vi "TSCAN_Table.vi"(6 "Message Name":string[][](array[string]), 7 "ms?":bool, 8 "SigValue":dbl[][](array[numeric]), 9 "SigName":string[][](array[string]), 10 "Buffer":T1(array[cluster]), 11 "MCListbox reference handle":refnum<vi>) -> ()   [LabVIEW 2014]
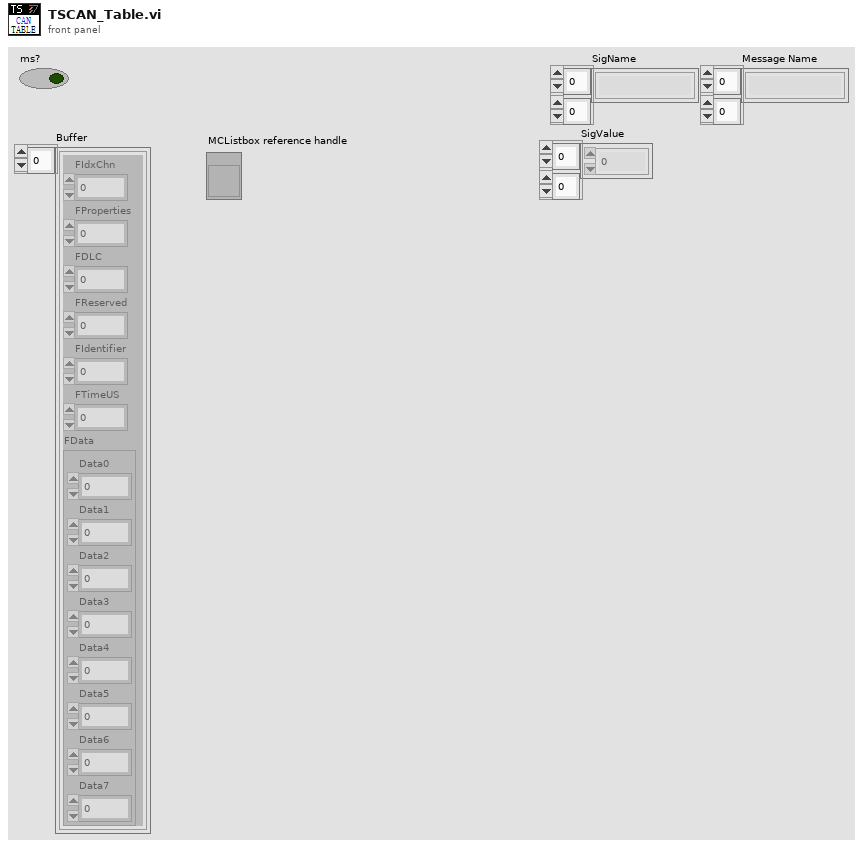
[diagram p1: front panel]
types:
  T1 = cluster{"FIdxChn":u8, "FProperties":u8, "FDLC":u8, "FReserved":u8, "FIdentifier":i32, "FTimeUS":u64, "FData":cluster{"Data0":u8, "Data1":u8, "Data2":u8, "Data3":u8, "Data4":u8, "Data5":u8, "Data6":u8, "Data7":u8}}[]
  T2 = cluster{"Data0":u8, "Data1":u8, "Data2":u8, "Data3":u8, "Data4":u8, "Data5":u8, "Data6":u8, "Data7":u8}
  T3 = typedef "LVRowAndColumnUnsignedTypeDef.ctl" = cluster{"Row":u32, "Column":u32}
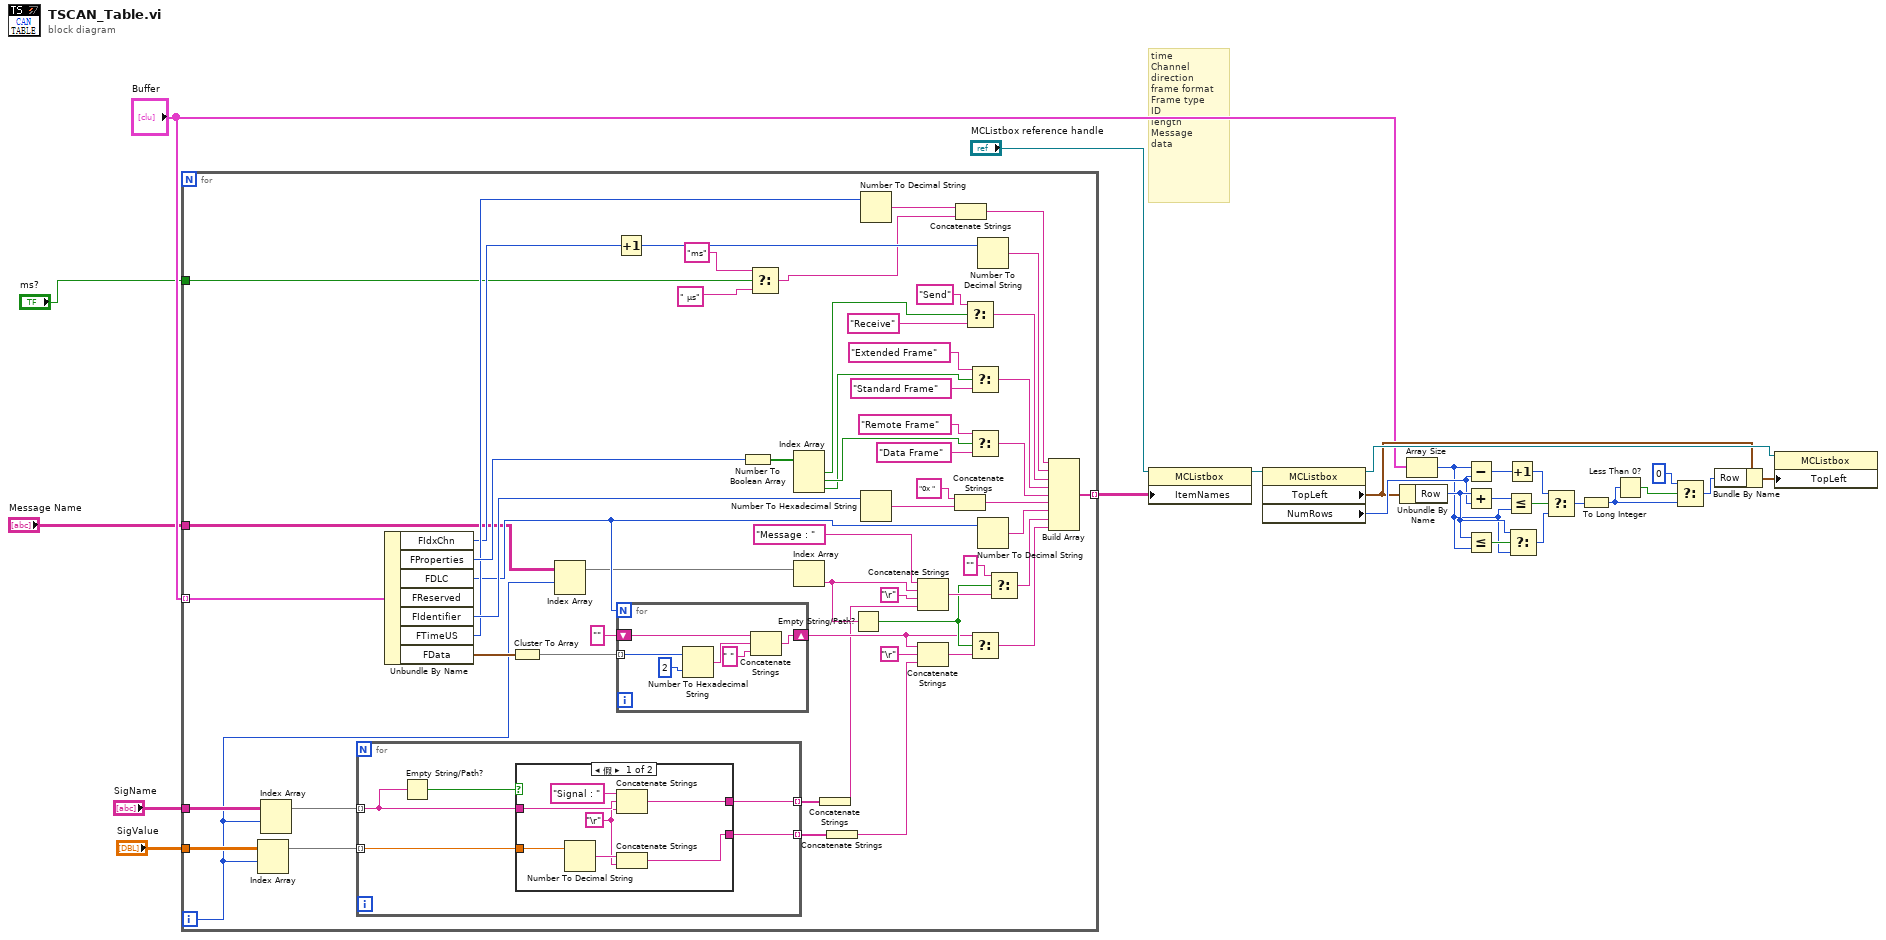
[diagram p0: block diagram]
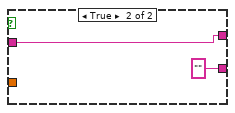
[diagram p2: hidden frame]
diagram:
  # "time\nChannel\ndirection\nframe format\nFrame type\nID\nlength\nMessage\ndata"
  n1 = for {
    tunnel: "Buffer" -> [w82] mode=indexing
    tunnel: [w59] -> w25 mode=indexing
    tunnel: "Message Name" -> [w45]
    tunnel: "SigValue" -> [w44]
    tunnel: "SigName" -> [w43]
    tunnel: "ms?" -> [w26]
    i -> [w30]
    n2 = Index Array(array=w44, index (row)=w30) -> (element=w31:dbl[])  [unwired: 1 in]
    n3 = Index Array(array=w43, index (row)=w30) -> (element=w32:string[])  [unwired: 1 in]
    n4 = for {
      tunnel: w32 -> [w87] mode=indexing
      tunnel: [w86] -> w48 mode=indexing
      tunnel: w31 -> [w84] mode=indexing
      tunnel: [w83] -> w37 mode=indexing
      n5 = Empty String/Path?(string/path=w87) -> (empty?=w85:bool)
      n6 = case shown="假" w85 {
        tunnel: w87 -> [w94 w96]
        tunnel: [w93 w96] -> w86
        tunnel: w84 -> [w91 _]
        tunnel: [w88 ""] -> w83
        frame False {
          w89 = "\r"
          n7 = Number To Decimal String(number=w91) -> (decimal integer string=w90:string)  [unwired: 1 in]
          n8 = Concatenate Strings("Signal : " ("字符串"), w94, w89) -> (w93:string)
          n9 = Concatenate Strings(w90, w89) -> (w88:string)
        }
        frame True {
        }
      }
    }
    n10 = Unbundle By Name(w82) -> ("FIdxChn"=w58:u8, "FProperties"=w81:u8, "FDLC"=w66:u8, "FIdentifier"=w70:i32, "FTimeUS"=w69:u64, "FData"=w67:T2)  [unwired: 1 out]
    n11 = Cluster To Array(cluster=w67) -> (array=w65:u8[])
    n12 = Index Array(array=w45, index (row)=w30) -> (element=w33:string[])  [unwired: 1 in]
    n13 = Increment(x=w58) -> (x+1=w57:u8)
    n14 = for {
      N: w66 -> [_]
      tunnel: w65 -> [w99] mode=indexing
      shift-right: [w101] -> w39
      shift-left: "" -> [w102]
      n15 = Number To Hexadecimal String(1:i16 2 ("width (-)"), 2:w99) -> (0:w98:string)
      n16 = Concatenate Strings(w102, w98, " " ("string")) -> (w101:string)
    }
    n17 = Number To Boolean Array(number=w81) -> (Boolean array=w80:bool[])
    n18 = Select(t="ms" ("字符串"), s=w26, f=" μs" ("字符串")) -> (s? t:f=w27:string)
    n19 = Index Array(array=w80) -> (element #1=w79:bool, element #2=w74:bool, element #3=w71:bool)  [unwired: 3 in]
    n20 = Index Array(array=w33) -> (element=w50:string)  [unwired: 1 in]
    n21 = Concatenate Strings(w48) -> (w35:string)
    n22 = Concatenate Strings(w37) -> (w34:string)
    n23 = Empty String/Path?(string/path=w50) -> (empty?=w40:bool)
    n24 = Number To Decimal String(number=w69) -> (decimal integer string=w52:string)  [unwired: 1 in]
    n25 = Number To Hexadecimal String(2:w70) -> (0:w55:string)  [unwired: 1 in]
    n26 = Concatenate Strings("Message : " ("字符串"), w50, "\r", w35) -> (w47:string)
    n27 = Concatenate Strings(w39, "\r", w34) -> (w42:string)
    n28 = Concatenate Strings("0x " ("字符串"), w55) -> (w56:string)
    n29 = Concatenate Strings(w52, w27) -> (w53:string)
    n30 = Select(t="Send", s=w79, f="Receive") -> (s? t:f=w63:string)
    n31 = Select(t="Extended Frame", s=w71, f="Standard Frame") -> (s? t:f=w62:string)
    n32 = Select(t="Remote Frame", s=w74, f="Data Frame") -> (s? t:f=w61:string)
    n33 = Select(t=w39, s=w40, f=w42) -> (s? t:f=w38:string)
    n34 = Number To Decimal String(number=w57) -> (decimal integer string=w64:string)  [unwired: 1 in]
    n35 = Number To Decimal String(number=w66) -> (decimal integer string=w60:string)  [unwired: 1 in]
    n36 = Select(t="", s=w40, f=w47) -> (s? t:f=w36:string)
    n37 = Build Array(w53, w64, w63, w62, w61, w56, w60, w36, w38) -> (w59:string[])
  }
  n38 = property class="MCListbox"(reference="MCListbox reference handle", "ItemNames"=w25) -> (reference out=w6:refnum<vi>)  [unwired: 1 in, 1 out]
  n39 = property class="MCListbox"(reference=w6) -> (reference out=w14:refnum<vi>, "TopLeft"=w13:T3, "NumRows"=w21:u32)  [unwired: 1 in, 1 out]
  n40 = Unbundle By Name(w13) -> ("Row"=w22:u32)
  n41 = Array Size(array="Buffer") -> (size(s)=w19:i32)
  n42 = Subtract(x=w19, y=w21) -> (x-y=w18:u32)
  n43 = Add(x=w22, y=w21) -> (x+y=w20:u32)
  n44 = Less Or Equal?(x=w22, y=w19) -> (x <= y?=w23:bool)
  n45 = Less Or Equal?(x=w20, y=w19) -> (x <= y?=w15:bool)
  n46 = Increment(x=w18) -> (x+1=w16:u32)
  n47 = Select(t=w22, s=w23, f=w19) -> (s? t:f=w17:u32)
  n48 = Select(t=w16, s=w15, f=w17) -> (s? t:f=w12:u32)
  n49 = To Long Integer(number=w12) -> (32bit integer=w10:i32)
  n50 = Less Than 0?(x=w10) -> (x < 0?=w11:bool)
  n51 = Select(t=0, s=w11, f=w10) -> (s? t:f=w9:i32)
  n52 = Bundle By Name(cluster=w13, "Row"=w9) -> (w7:T3)
  n53 = property class="MCListbox"(reference=w14, "TopLeft"=w7) -> ()  [unwired: 1 in, 2 out]
